vi "Actor Core.vi"(8 "error in":errorcluster, 11 "New Project Wizard in":refnum<class "New Project Wizard.lvclass">) -> (0 "error out":errorcluster, 3 "Actor out":refnum<class "Actor.lvclass">)   [LabVIEW 2013, in "SET Project Editor.lvlib" / "New Project Wizard.lvclass"]
doc: "(<B>Filename</B>: Actor Framework.lvlib:Actor.lvclass:Actor Core.vi)\n\nReceives messages to the actor, reacts to them, and initiates any error handling that may shut the actor down.\n\nDescendant classes may override this VI to append parallel tasks for the actor to complete while it handles messages. Overrides use the Call Parent Method node."
uses:
  New Project Wizard.lvclass
  <vilib>/ActorFramework/Actor/Actor.lvclass
  <vilib>/ActorFramework/Actor/Actor.lvclass/Actor.ctl
  <vilib>/ActorFramework/Message Enqueuer/Message Enqueuer.lvclass/Message Enqueuer.ctl
  New Project Wizard.lvclass/New Project Wizard.ctl
  lib/printf/messages/General/LV_Printf Msg.lvclass/LV_Printf Msg.ctl
  UI Wizard/UI Wizard.lvclass
  lib/printf/messages/General/Read Message.vi
  <vilib>/ActorFramework/Message Enqueuer/Init from Existing Queue.vi
  <vilib>/ActorFramework/Message Enqueuer/Enqueue.vi
  <vilib>/ActorFramework/Message Priority Queue/Priority Enqueue.vi
  <vilib>/ActorFramework/Message Enqueuer/Message Enqueuer.lvclass
  <vilib>/ActorFramework/Stop Msg/Stop Msg.lvclass
  UI Wizard Messages/Extract Project Strings Msg/Extract Project Strings Msg.lvclass
  UI Wizard Messages/Apply Changes Msg/Apply Changes Msg.lvclass
  lib/printf/Core/LV_Printf Core.lvclass
  lib/printf/messages/General/LV_Printf Msg.lvclass
panel:
  in  "Tab Control":enum32{"Page 1", "Page 2"}(tab)
  in  "Next1":bool
  out "ProjectName":string
  in  "Cancel1":bool
  in  "Default Language":string(combo)="en"
  in  "VI Selector":i32(listbox)
  in  "RTM Selector":i32(listbox)
  out "Status":string
  in  "Prev2":bool
  in  "Finish":bool
  in  "Cancel2":bool
  # "New Project Wizard"
  # "Select VIs"
  # "Select Run-Time Menus"
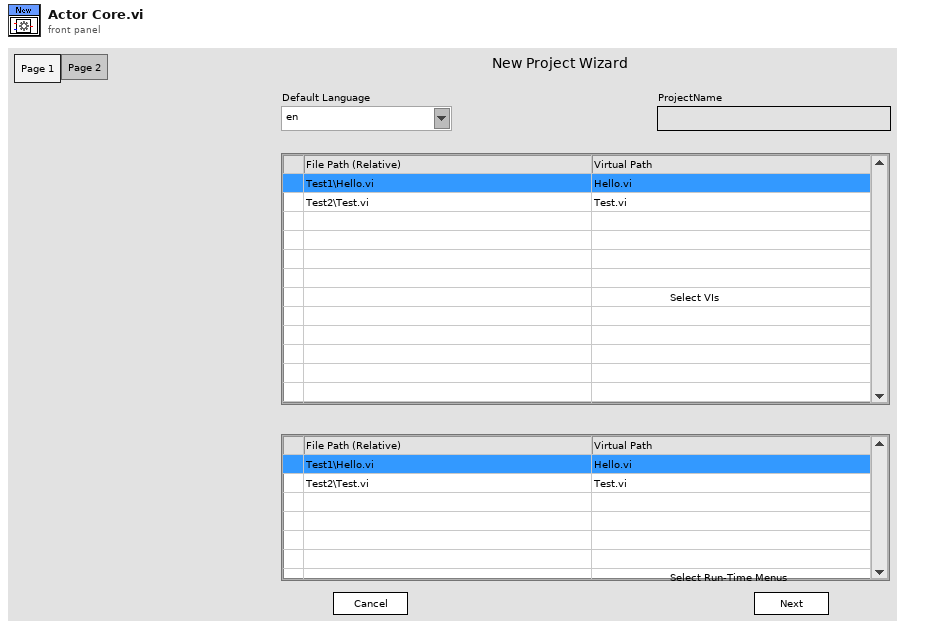
[diagram p1: front panel]
types:
  T1 = typedef "LVPoint32TypeDef.ctl" = cluster{"Horizontal":i32, "Vertical":i32}
  T2 = typedef "LVRowAndColumnTypeDef.ctl" = cluster{"Row":i32, "Column":i32}
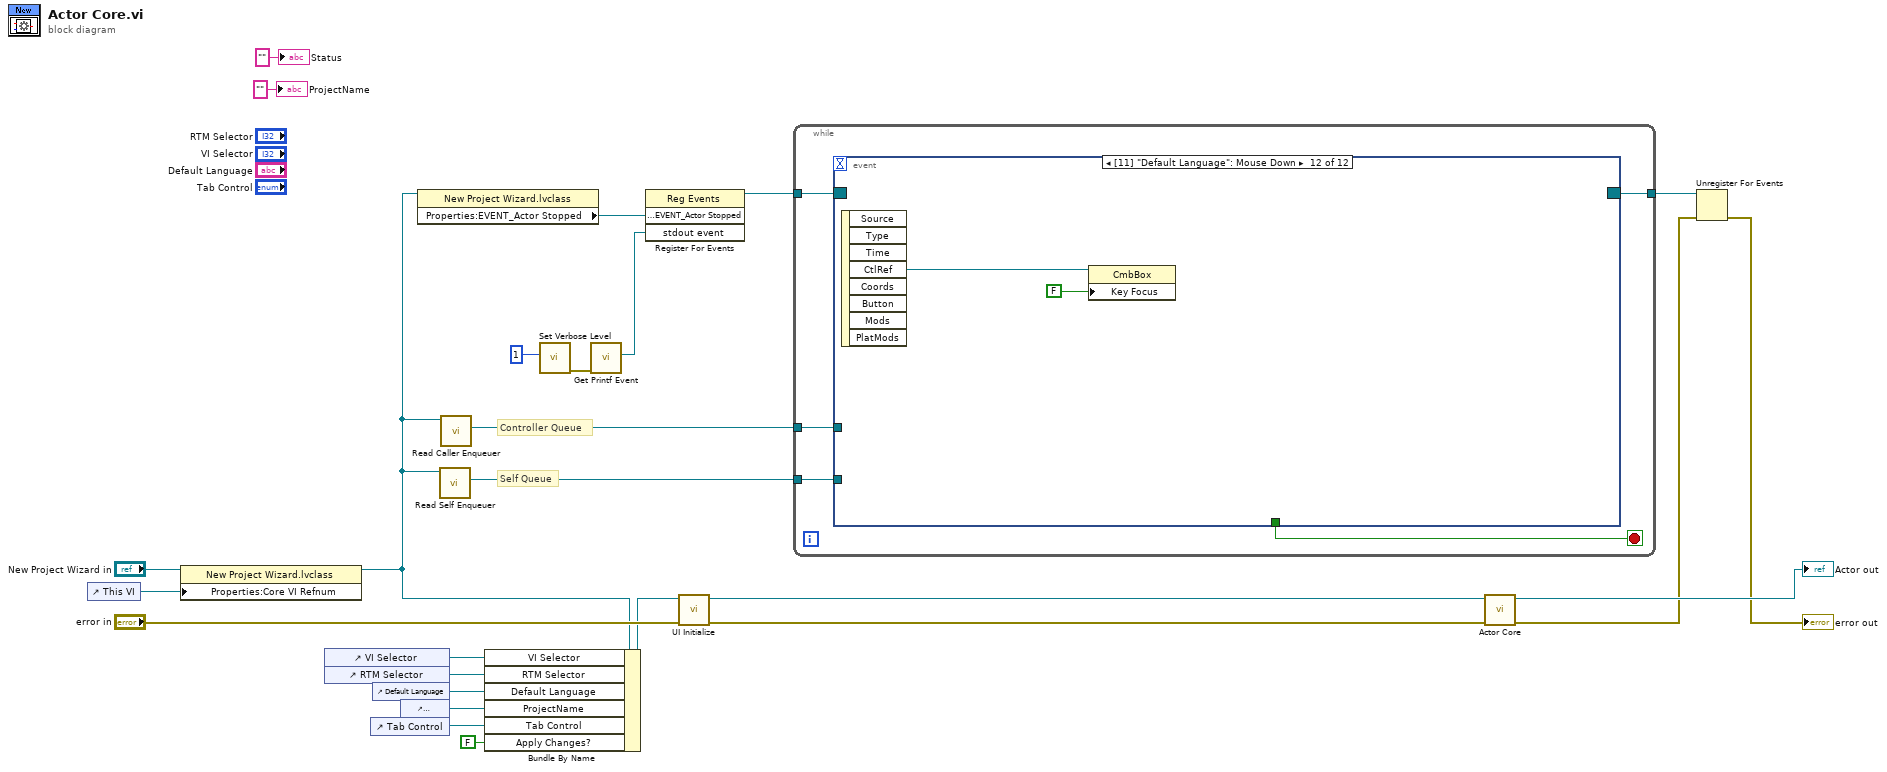
[diagram p0: block diagram]
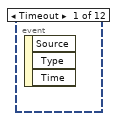
[diagram p2: hidden frame]
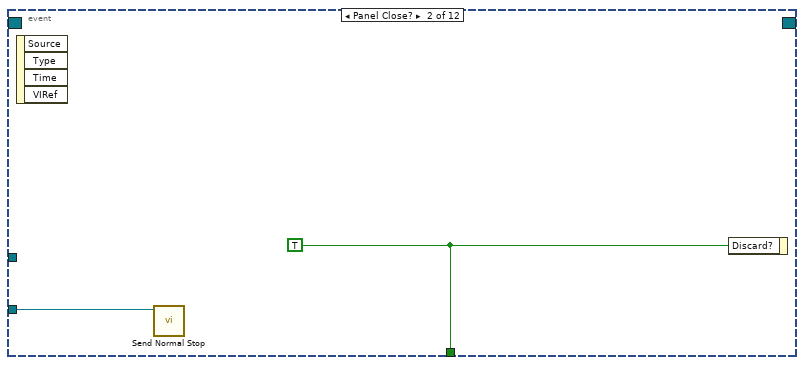
[diagram p3: hidden frame]
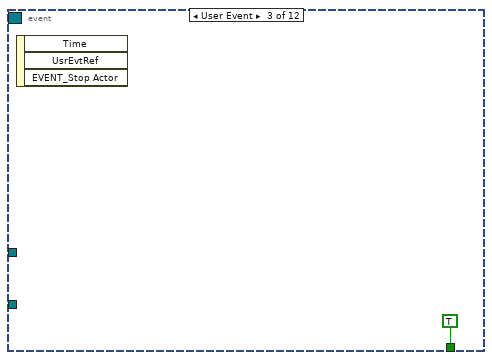
[diagram p4: hidden frame]
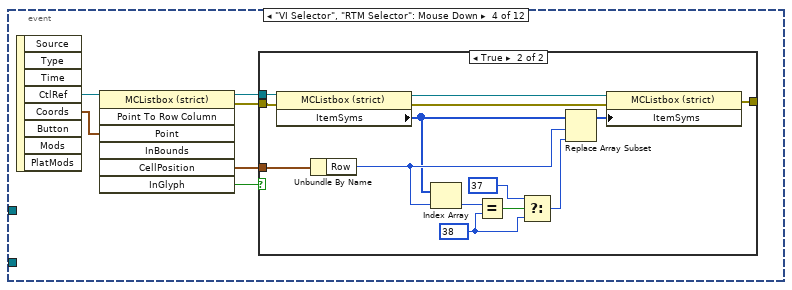
[diagram p5: hidden frame]
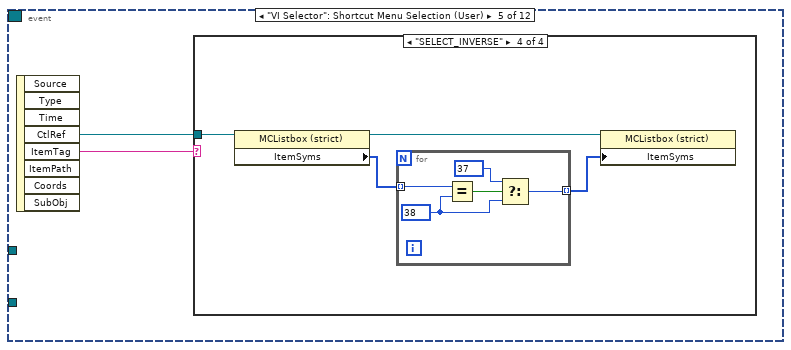
[diagram p7: hidden frame]
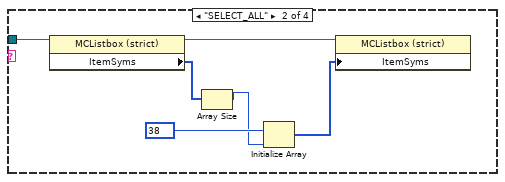
[diagram p9: hidden frame]
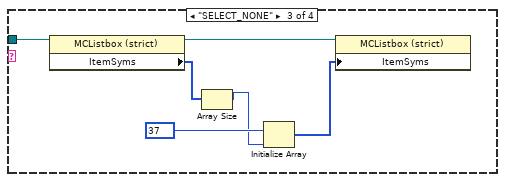
[diagram p10: hidden frame]
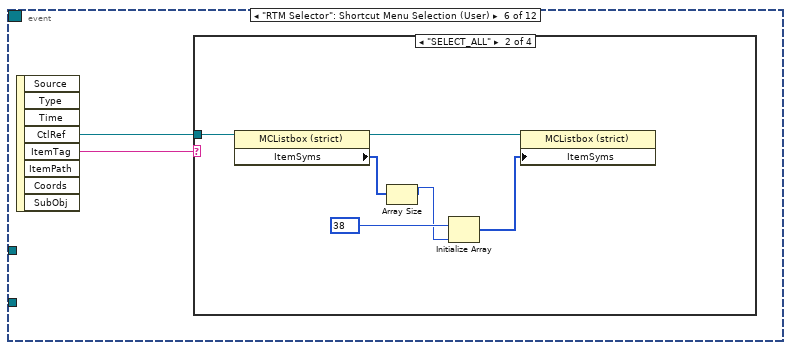
[diagram p11: hidden frame]
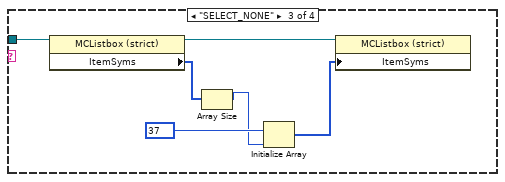
[diagram p13: hidden frame]
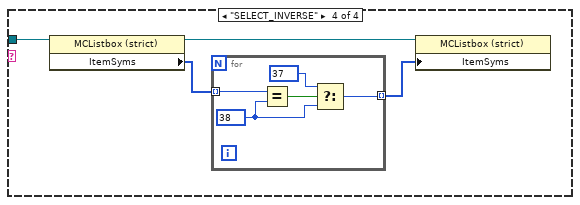
[diagram p14: hidden frame]
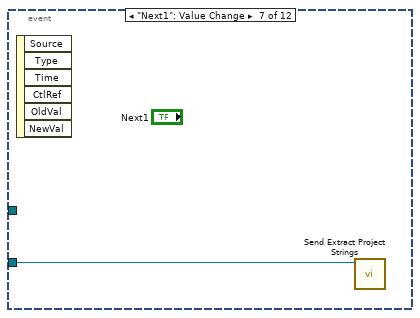
[diagram p15: hidden frame]
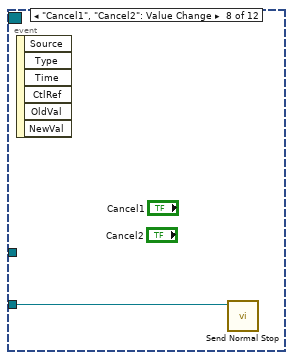
[diagram p16: hidden frame]
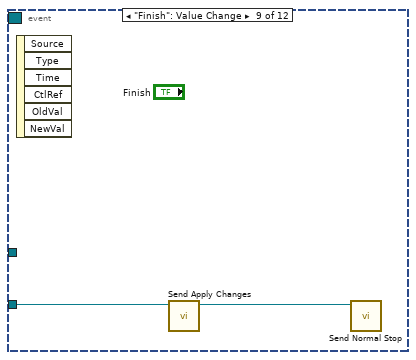
[diagram p17: hidden frame]
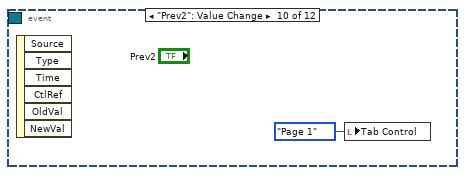
[diagram p18: hidden frame]
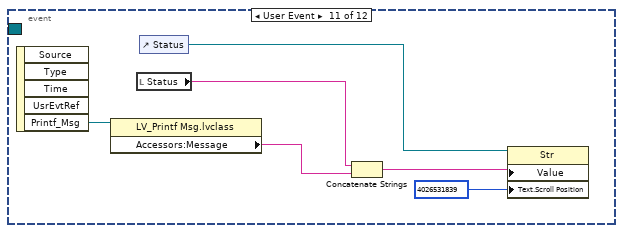
[diagram p19: hidden frame]
diagram:
  # "Controller Queue"
  # "Self Queue"
  n1 = control-ref of="This VI"() -> (w18:refnum<vi>)
  n2 = property class="New Project Wizard.lvclass"(reference="New Project Wizard in", "Properties:Core VI Refnum"=w18) -> (reference out=w10:refnum<class "New Project Wizard.lvclass">)  [unwired: 1 in, 1 out]
  n3 = control-ref of="VI Selector"() -> (w8:refnum<vi>)
  n4 = control-ref of="RTM Selector"() -> (w7:refnum<vi>)
  n5 = control-ref of="Tab Control"() -> (w5:refnum<vi>)
  n6 = control-ref of="Default Language"() -> (w1:refnum<vi>)
  n7 = control-ref of="ProjectName"() -> (w6:refnum<vi>)
  n8 = property class="New Project Wizard.lvclass"(reference=w10) -> ("Properties:EVENT_Actor Stopped"=w25:refnum<user-event>)  [unwired: 1 in, 2 out]
  n9 = call <vilib>:"Read Self Enqueuer.vi"("Actor"=w10) -> ("Self Enqueuer"=w23:refnum<class "Message Enqueuer.lvclass">)  [unwired: 10 in]
  n10 = call <vilib>:"Read Caller Enqueuer.vi"("Actor"=w10) -> ("Caller Enqueuer"=w24:refnum<class "Message Enqueuer.lvclass">)  [unwired: 10 in]
  n11 = Bundle By Name(cluster=w10, "VI Selector"=w8, "RTM Selector"=w7, "Default Language"=w1, "ProjectName"=w6, "Tab Control"=w5, "Apply Changes?"=FALSE) -> (w9:refnum<class "New Project Wizard.lvclass">)
  n12 = call "Set Verbose Level.vi"("Verbose Level"=1) -> ("error out"=w12:errorcluster)  [unwired: 10 in]
  n13 = call "Get Printf Event.vi"("error in (no error)"=w12) -> ("stdout event"=w11:refnum<user-event>)  [unwired: 8 in, 2 out]
  n14 = register-events(w25, w11) -> (reference out=w13:refnum<event-registration>)  [unwired: 2 in, 1 out]
  n15 = call-dynamic "UI Initialize.vi"("error in (no error)"="error in", "New Project Wizard in"=w9) -> ("error out"=w16:errorcluster, "New Project Wizard out"=w17:refnum<class "New Project Wizard.lvclass">)  [unwired: 8 in]
  n16 = while {
    tunnel: w13 -> [w30]
    tunnel: [w29] -> w22
    tunnel: w23 -> [w28]
    tunnel: w24 -> [w27]
    stop <- w31 stop-if-true
    n17 = event shown="[11] \"Default Language\": Mouse Down" {
      selector: w30 -> [_ _ _ _ _ _ _ _ _ _ _ _]
      dyn-events: [_ _ _ _ _ _ _ _ _ _ _ _] -> w29
      timeout: _ -> [_ _ _ _ _ _ _ _ _ _ _ _]
      tunnel: [_ w33 TRUE ("Discard?") _ _ _ _ _ _ _ _ _] -> w31
      tunnel: w28 -> [_ w32 _ _ _ _ w102 w103 w105 _ _ _]
      tunnel: w27 -> [_ _ _ _ _ _ _ _ _ _ _ _]
      event Timeout {
        n18 = event-data() -> ()  [unwired: 1 in, 3 out]
      }
      event Panel Close? {
        w33 = TRUE ("Discard?")
        n19 = event-data() -> ()  [unwired: 1 in, 4 out]
        n20 = call <vilib>:"Send Normal Stop.vi"("Message Enqueuer"=w32) -> ()  [unwired: 10 in, 1 out]
        n21 = event-data("Discard?"=w33) -> ()  [unwired: 1 in, 1 out]
      }
      event User Event {
        n22 = event-data() -> ()  [unwired: 1 in, 3 out]
      }
      event "VI Selector", "RTM Selector": Mouse Down {
        n23 = event-data() -> ("CtlRef"=w36:refnum<vi>, "Coords"=w35:T1)  [unwired: 1 in, 6 out]
        n24 = invoke class="MCListbox (strict)" method="Point To Row Column"(reference=w36, "Point"=w35) -> (reference out=w38:refnum<vi>, error out=w39:errorcluster, "CellPosition"=w40:T2, "InGlyph"=w37:bool)  [unwired: 5 in, 3 out]
        n25 = case shown="True" w37 {
          tunnel: w40 -> [_ w55]
          tunnel: w39 -> [w41 w54]
          tunnel: [w41 w51] -> _
          tunnel: w38 -> [_ w50]
          frame False {
          }
          frame True {
            w46 = 38
            n26 = property on="Property Node" class="MCListbox (strict)"(reference=w50, error in=w54) -> (reference out=w49:refnum<vi>, error out=w53:errorcluster, "ItemSyms"=w43:i32[])
            n27 = Unbundle By Name(w55) -> ("Row"=w44:i32)
            n28 = Index Array(array=w43, index=w44) -> (element=w48:i32)
            n29 = Equal?(x=w48, y=w46) -> (x = y?=w47:bool)
            n30 = Select(t=37, s=w47, f=w46) -> (s? t:f=w45:i32)
            n31 = Replace Array Subset(array=w43, new element=w45, index=w44) -> (w52:i32[])
            n32 = property on="Property Node" class="MCListbox (strict)"(reference=w49, error in=w53, "ItemSyms"=w52) -> (error out=w51:errorcluster)  [unwired: 1 out]
          }
        }
      }
      event "VI Selector": Shortcut Menu Selection (User) {
        n33 = event-data() -> ("CtlRef"=w56:refnum<vi>, "ItemTag"=w57:string)  [unwired: 1 in, 6 out]
        n34 = case shown="\"SELECT_INVERSE\"" w57 {
          tunnel: w56 -> [_ w63 w69 w73]
          frame "False", Default {
          }
          frame "SELECT_ALL" {
            n35 = property class="MCListbox (strict)"(reference=w63) -> (reference out=w58:refnum<vi>, "ItemSyms"=w62:i32[])  [unwired: 1 in, 1 out]
            n36 = Array Size(array=w62) -> (size(s)=w60:i32)
            n37 = Initialize Array(38, w60) -> (w59:i32[])
            n38 = property class="MCListbox (strict)"(reference=w58, "ItemSyms"=w59) -> ()  [unwired: 1 in, 2 out]
          }
          frame "SELECT_NONE" {
            n39 = property class="MCListbox (strict)"(reference=w69) -> (reference out=w64:refnum<vi>, "ItemSyms"=w68:i32[])  [unwired: 1 in, 1 out]
            n40 = Array Size(array=w68) -> (size(s)=w66:i32)
            n41 = Initialize Array(37, w66) -> (w65:i32[])
            n42 = property class="MCListbox (strict)"(reference=w64, "ItemSyms"=w65) -> ()  [unwired: 1 in, 2 out]
          }
          frame "SELECT_INVERSE" {
            n43 = property class="MCListbox (strict)"(reference=w73) -> (reference out=w72:refnum<vi>, "ItemSyms"=w71:i32[])  [unwired: 1 in, 1 out]
            n44 = for {
              tunnel: w71 -> [w78] mode=indexing
              tunnel: [w74] -> w70 mode=indexing
              w75 = 38
              n45 = Equal?(x=w78, y=w75) -> (x = y?=w77:bool)
              n46 = Select(t=37, s=w77, f=w75) -> (s? t:f=w74:i32)
            }
            n47 = property class="MCListbox (strict)"(reference=w72, "ItemSyms"=w70) -> ()  [unwired: 1 in, 2 out]
          }
        }
      }
      event "RTM Selector": Shortcut Menu Selection (User) {
        n48 = event-data() -> ("CtlRef"=w79:refnum<vi>, "ItemTag"=w80:string)  [unwired: 1 in, 6 out]
        n49 = case shown="\"SELECT_ALL\"" w80 {
          tunnel: w79 -> [_ w86 w92 w96]
          frame "False", Default {
          }
          frame "SELECT_ALL" {
            n50 = property class="MCListbox (strict)"(reference=w86) -> (reference out=w81:refnum<vi>, "ItemSyms"=w85:i32[])  [unwired: 1 in, 1 out]
            n51 = Array Size(array=w85) -> (size(s)=w83:i32)
            n52 = Initialize Array(38, w83) -> (w82:i32[])
            n53 = property class="MCListbox (strict)"(reference=w81, "ItemSyms"=w82) -> ()  [unwired: 1 in, 2 out]
          }
          frame "SELECT_NONE" {
            n54 = property class="MCListbox (strict)"(reference=w92) -> (reference out=w87:refnum<vi>, "ItemSyms"=w91:i32[])  [unwired: 1 in, 1 out]
            n55 = Array Size(array=w91) -> (size(s)=w89:i32)
            n56 = Initialize Array(37, w89) -> (w88:i32[])
            n57 = property class="MCListbox (strict)"(reference=w87, "ItemSyms"=w88) -> ()  [unwired: 1 in, 2 out]
          }
          frame "SELECT_INVERSE" {
            n58 = property class="MCListbox (strict)"(reference=w96) -> (reference out=w95:refnum<vi>, "ItemSyms"=w94:i32[])  [unwired: 1 in, 1 out]
            n59 = for {
              tunnel: w94 -> [w101] mode=indexing
              tunnel: [w97] -> w93 mode=indexing
              w98 = 38
              n60 = Equal?(x=w101, y=w98) -> (x = y?=w100:bool)
              n61 = Select(t=37, s=w100, f=w98) -> (s? t:f=w97:i32)
            }
            n62 = property class="MCListbox (strict)"(reference=w95, "ItemSyms"=w93) -> ()  [unwired: 1 in, 2 out]
          }
        }
      }
      event "Next1": Value Change {
        n63 = event-data() -> ()  [unwired: 1 in, 6 out]
        n64 = call "Send Extract Project Strings.vi"("Message Enqueuer"=w102) -> ()  [unwired: 9 in, 2 out]
      }
      event "Cancel1", "Cancel2": Value Change {
        n65 = event-data() -> ()  [unwired: 1 in, 6 out]
        n66 = call <vilib>:"Send Normal Stop.vi"("Message Enqueuer"=w103) -> ()  [unwired: 10 in, 1 out]
      }
      event "Finish": Value Change {
        n67 = event-data() -> ()  [unwired: 1 in, 6 out]
        n68 = call "Send Apply Changes.vi"("Message Enqueuer"=w105) -> ("Message Enqueuer out"=w104:refnum<class "Message Enqueuer.lvclass">)  [unwired: 9 in, 1 out]
        n69 = call <vilib>:"Send Normal Stop.vi"("Message Enqueuer"=w104) -> ()  [unwired: 10 in, 1 out]
      }
      event "Prev2": Value Change {
        n70 = event-data() -> ()  [unwired: 1 in, 6 out]
        n71 = local write "Tab Control"(enum32{"Page 1", "Page 2"}."Page 1" ("Tab Control")) -> ()
      }
      event User Event {
        n72 = event-data() -> ("Printf_Msg"=w110:refnum<class "LV_Printf Msg.lvclass">)  [unwired: 1 in, 4 out]
        n73 = property class="LV_Printf Msg.lvclass"(reference=w110) -> ("Accessors:Message"=w108:string)  [unwired: 1 in, 2 out]
        n74 = local read "Status"() -> (w109:string)
        n75 = control-ref of="Status"() -> (w112:refnum<vi>)
        n76 = Concatenate Strings(w109, w108) -> (w107:string)
        n77 = property class="Str"(reference=w112, "Value"=w107, "Text.Scroll Position"=u32 4026531839) -> ()  [unwired: 1 in, 2 out]
      }
      event "Default Language": Mouse Down {
        n78 = event-data() -> ("CtlRef"=w114:refnum<vi>)  [unwired: 1 in, 7 out]
        n79 = property class="CmbBox"(reference=w114, "Key Focus"=FALSE) -> ()  [unwired: 1 in, 2 out]
      }
    }
  }
  n80 = call-parent "Actor Core.vi"("error in"=w16, "Actor in"=w17) -> ("error out"=w21:errorcluster, "Actor out"=→"Actor out":refnum<class "Actor.lvclass">)  [unwired: 8 in]
  n81 = Unregister For Events(event registration refnum=w22, error in=w21) -> (error out=→"error out":errorcluster)
  "ProjectName" <- "" ("ProjectName")
  "Status" <- "" ("Status")
